vi "MapaIntensidade-FROG.vi"() -> ()   [LabVIEW 2014]
doc: "Mapa de Intensidade FROG\n\nAndré Romero - 2022\nandretec@ifsc.usp.br"
uses:
  FROG-GlobalVar.vi
panel:
  out "Intensity Graph":dbl[][](graph)
  out "Numeric 2":i32
  out "Numeric":i32=4
  out "appended array":dbl[](array[numeric])
  out "Progresso":i32=4
  out "size(s) 2":i32[](array[numeric])=[5, 5]
  out "Array":dbl[][](array[numeric])=[[222.8, 222.8, 222.8, 221.0, 0.0], [220.2, 220.7, 221.6, 222.2, 222.3], [222.4, 222.4, 222.4, 222.5, 0.0], [222.5, 222.5, 222.5, 222.5, 222.5], [0.0, 0.0, 0.0, 0.0, 0.0]]
  out "GO":bool
  out "Temporal FWHM":dbl
  in  "milliseconds to wait":u32=500
  out "size(s)":i32
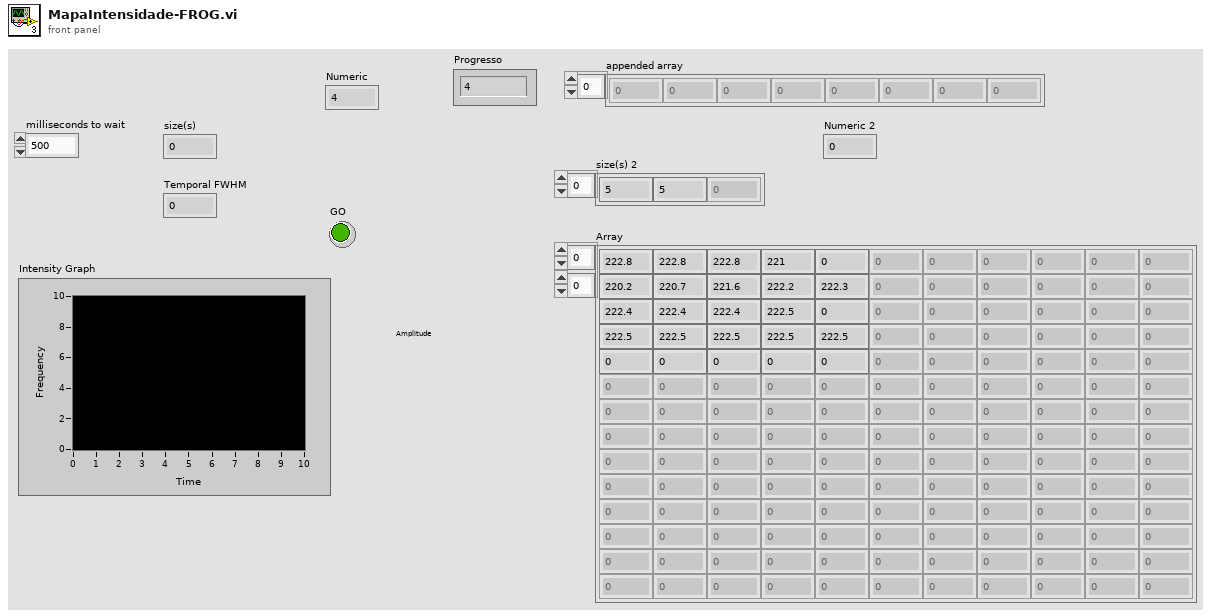
[diagram p1: front panel]
types:
  T1 = typedef "FROG.ctl" = cluster{"Delay increment":dbl, "Center Wavelength":dbl, "Frog Error was":dbl, "Temporal FWHM":dbl, "Spectral FWHM":dbl, "FWHM Time-Bandwidth Product":dbl, "RMS Time-Bandwidth Product":dbl}
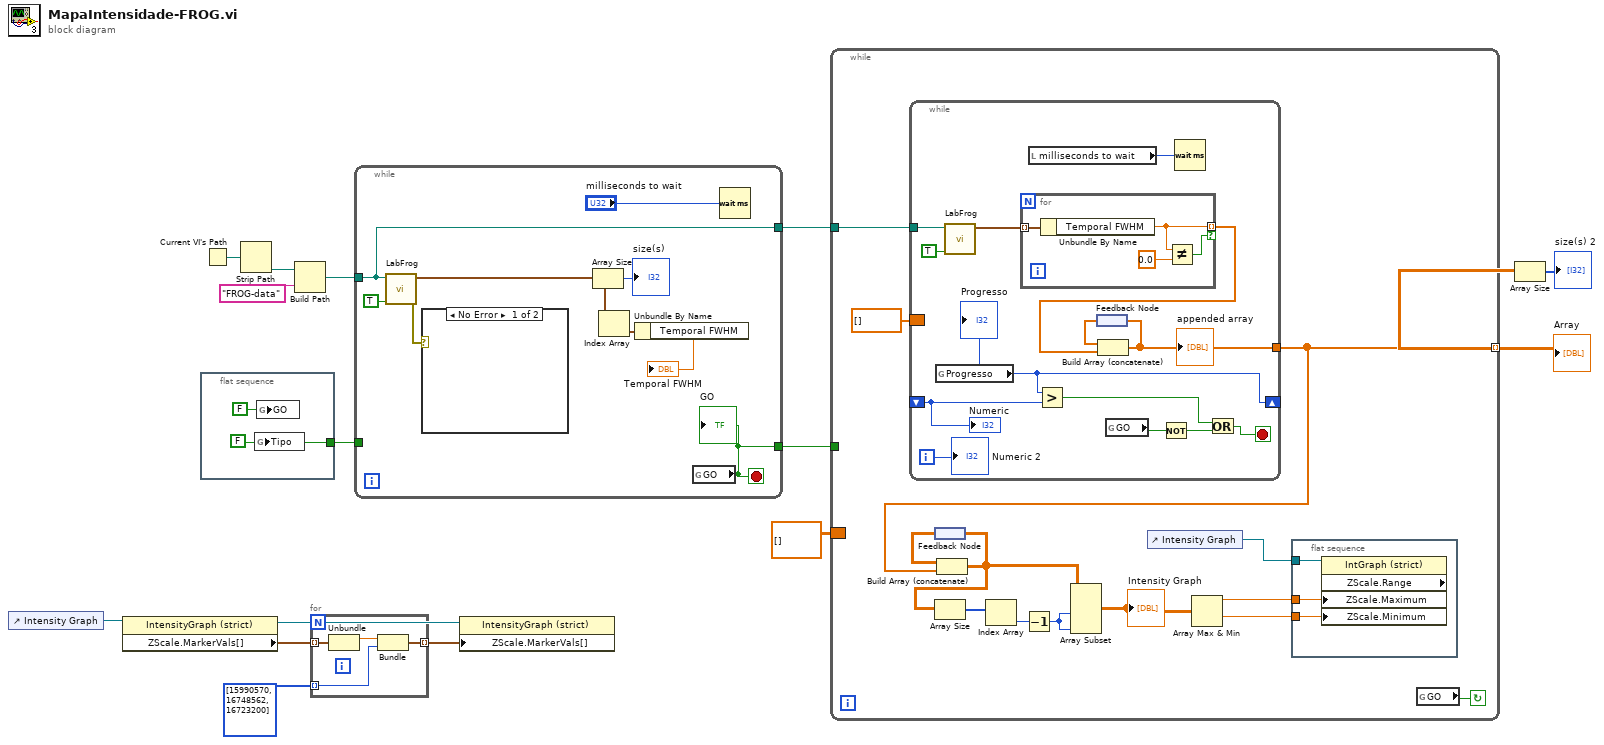
[diagram p0: block diagram]
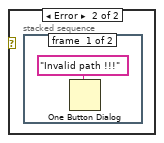
[diagram p2: hidden frame]
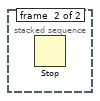
[diagram p3: hidden frame]
diagram:
  n1 = control-ref of="Intensity Graph"() -> (w2:refnum<vi>)
  n2 = property on="Property Node" class="IntensityGraph (strict)"(reference=w2) -> (reference out=w3:refnum<vi>, "ZScale.MarkerVals[]"=w6:cluster{dbl, u32}[])  [unwired: 1 in, 1 out]
  n3 = flat-sequence {
    tunnel: [w16] -> w11
    frame #0 {
      w16 = FALSE ("Tipo")
      n4 = global write "FROG-GlobalVar.vi" "Tipo"(w16) -> ()
      n5 = global write "FROG-GlobalVar.vi" "GO"(FALSE ("GO")) -> ()
    }
  }
  n6 = Current VI's Path() -> (path=w15:path)
  n7 = Strip Path(path=w15) -> (stripped path=w13:path)  [unwired: 1 out]
  n8 = Build Path(base path=w13, name or relative path="FROG-data") -> (appended path=w12:path)
  n9 = for {
    tunnel: w6 -> [w21] mode=indexing
    tunnel: u32[] [15990570, 16748562, 16723200] ("Custom Marker Colors") -> [w19] mode=indexing
    tunnel: [w18] -> w4 mode=indexing
    n10 = Unbundle(w21) -> (w20:dbl)  [unwired: 1 out]
    n11 = Bundle(w20, "Color Box"=w19) -> (w18:cluster{dbl, "Color Box":u32})  [unwired: 1 in]
  }
  n12 = while {
    tunnel: w12 -> [w25]
    tunnel: w11 -> [_]
    tunnel: [w26] -> w10
    tunnel: [w25] -> w9
    stop <- w26 stop-if-true
    n13 = call "LabFrog.vi"("Simutation"=TRUE, "FROG path"=w25) -> ("error out"=w23:errorcluster, "FROG data"=w28:T1[])  [unwired: 8 in]
    n14 = case shown="No Error" w23 {
      frame No Error {
      }
      frame Error {
        n15 = stacked-sequence {
          frame #0 {
            n16 = One Button Dialog(message="Invalid path !!!") -> ()  [unwired: 1 in, 1 out]
          }
          frame #1 {
            n17 = Stop() -> ()  [unwired: 1 in]
          }
        }
      }
    }
    n18 = Array Size(array=w28) -> (size(s)=→"size(s)":i32)
    n19 = Index Array(array=w28) -> (element=w27:T1)  [unwired: 1 in]
    n20 = Unbundle By Name(w27) -> ("Temporal FWHM"=→"Temporal FWHM":dbl)
    n21 = global read "FROG-GlobalVar.vi" "GO"() -> (w26:bool)
    "GO" <- w26
    n22 = Wait (ms)(milliseconds to wait="milliseconds to wait") -> ()  [unwired: 1 out]
  }
  n23 = property on="Property Node" class="IntensityGraph (strict)"(reference=w3, "ZScale.MarkerVals[]"=w4) -> ()  [unwired: 1 in, 2 out]
  n24 = while {
    tunnel: w10 -> [_]
    tunnel: w9 -> [w44]
    tunnel: [w40] -> w1 mode=indexing
    border: dbl[][] [] -> [_]
    stop <- w43 continue-if-true
    n25 = while {
      tunnel: w44 -> [w61]
      border: dbl[] [] -> [_]
      shift-right: [w53] -> _
      shift-left: _ -> [w50]
      tunnel: [w54] -> w40
      i -> [w49]
      stop <- w57 stop-if-true
      n26 = global read "FROG-GlobalVar.vi" "Progresso"() -> (w53:i32)
      "Progresso" <- w53
      n27 = call "LabFrog.vi"("Simutation"=TRUE, "FROG path"=w61) -> ("FROG data"=w52:T1[])  [unwired: 8 in, 1 out]
      n28 = for {
        tunnel: w52 -> [w65] mode=indexing
        tunnel: [w62] -> w58 mode=indexing if=w64
        n29 = Unbundle By Name(w65) -> ("Temporal FWHM"=w62:dbl)
        n30 = Not Equal?(x=w62, y=0.0) -> (x != y?=w64:bool)
      }
      n31 = local read "milliseconds to wait"() -> (w60:u32)
      n32 = Greater?(x=w53, y=w50) -> (0:w55:bool)
      n33 = feedback #1() -> (w59:dbl[])
      n34 = Build Array (concatenate)(w59, w58) -> (w54:dbl[])
      "appended array" <- w54
      n35 = feedback-in #1(w54) -> ()
      n36 = global read "FROG-GlobalVar.vi" "GO"() -> (w56:bool)
      n37 = Not(x=w56) -> (.not. x?=w51:bool)
      n38 = Wait (ms)(milliseconds to wait=w60) -> ()  [unwired: 1 out]
      n39 = Or(x=w55, y=w51) -> (x .or. y?=w57:bool)
      "Numeric" <- w50
      "Numeric 2" <- w49
    }
    n40 = feedback #2() -> (w41:dbl[][])
    n41 = Build Array (concatenate)(w41, w40) -> (w38:dbl[][])
    n42 = feedback-in #2(w38) -> ()
    n43 = Array Size(array=w38) -> (size(s)=w39:i32[])
    n44 = Index Array(array=w39) -> (element=w37:i32)  [unwired: 1 in]
    n45 = Decrement(x=w37) -> (x-1=w36:i32)
    n46 = Array Subset(array=w38, length (row)=w36, length (col)=w36) -> (w35:dbl[][])  [unwired: 2 in]
    "Intensity Graph" <- w35
    n47 = control-ref of="Intensity Graph"() -> (w32:refnum<vi>)
    n48 = Array Max & Min(array=w35) -> (max value=w34:dbl, min value=w33:dbl)  [unwired: 2 out]
    n49 = flat-sequence {
      tunnel: w34 -> [w47]
      tunnel: w33 -> [w46]
      tunnel: w32 -> [w45]
      frame #0 {
        n50 = property on="Property Node" class="IntGraph (strict)" props=["ZScale", "Range", "ZScale", "Maximum", "ZScale", "Minimum"](reference=w45, "ZScale.Maximum"=w47, "ZScale.Minimum"=w46) -> ()  [unwired: 1 in, 3 out]
      }
    }
    n51 = global read "FROG-GlobalVar.vi" "GO"() -> (w43:bool)
  }
  "Array" <- w1
  n52 = Array Size(array=w1) -> (size(s)=→"size(s) 2":i32[])
